vi "Auto Play Path.vi"(8 "Operation":T1, 9 "Auto Data":T13, 10 "Motors":T2 {"Radii (ft)"."Right Back Position" format="%.2f"; "Radii (ft)"."Right Front Position" format="%.2f"; "Radii (ft)"."Left Back Position" format="%.2f"; "Radii (ft)"."Left Front Position" format="%.2f"; "Pigeon2"."Type" items=["CAN"=352321536, "TalonSRX"=33554432]}) -> (0 "Auto Done?":bool)   [LabVIEW 2023]
uses:
  swerve-template/Type Definitions/Data/Robot Velocities.ctl
  swerve-template/Type Definitions/Hardware/Swerve Drives/(NEO-NEO-ThroughBore-Pigeon2) Swerve.ctl
  swerve-template/Type Definitions/Hardware/4 Motor Sets/(NEO & NEO 550) 4 Motor Set.ctl
  <vilib>/Rock Robotics/WPI/MotorControl/WPI_MotorControlDeviceRef.ctl
  <vilib>/Rock Robotics/WPI/MotorControl/WPI_MotorControlType.ctl
  <vilib>/Rock Robotics/SystemInterfaces/DIO/FPGA_DIOPWMChannel.ctl
  <vilib>/Rock Robotics/WPI/PWM/WPI_PWMDeadband.ctl
  <vilib>/Rock Robotics/SystemInterfaces/DIO/FPGA_DIOChannel.ctl
  <vilib>/Rock Robotics/WPI/ThirdParty/Phoenix-LabVIEW/Pigeon IMU/CTRE_PigeonIMU_DeviceRef.ctl
  <vilib>/Rock Robotics/WPI/ThirdParty/Phoenix-LabVIEW/Pigeon IMU/CTRE_PigeonIMU_ConnectionType.ctl
  swerve-template/Type Definitions/Data/Pod Positions.ctl
  Implementation/Drive Operations.ctl
  <vilib>/Platform/TimedLoop/XDataNode/timing_clust.ctl
  <vilib>/Platform/TimedLoop/XDataNode/nitl_modes.ctl
  <vilib>/Platform/TimedLoop/XDataNode/wakeup.ctl
  <vilib>/Rock Robotics/WPI/ThirdParty/REV Robotics/REVLib/Typedef/Spark MAX Control Type.ctl
  <vilib>/Rock Robotics/WPI/DriverStation/WPI_DriverStationRobotMode2.ctl
  <vilib>/Rock Robotics/Network Tables/NT Read Boolean.vi
  Framework/Robot Global Data.vi
  <vilib>/Platform/TimedLoop/XDataNode/XDataNode.xnode
  <vilib>/Platform/TimedLoop/XDataNode/XDNodeRunTimeDep.lvlib
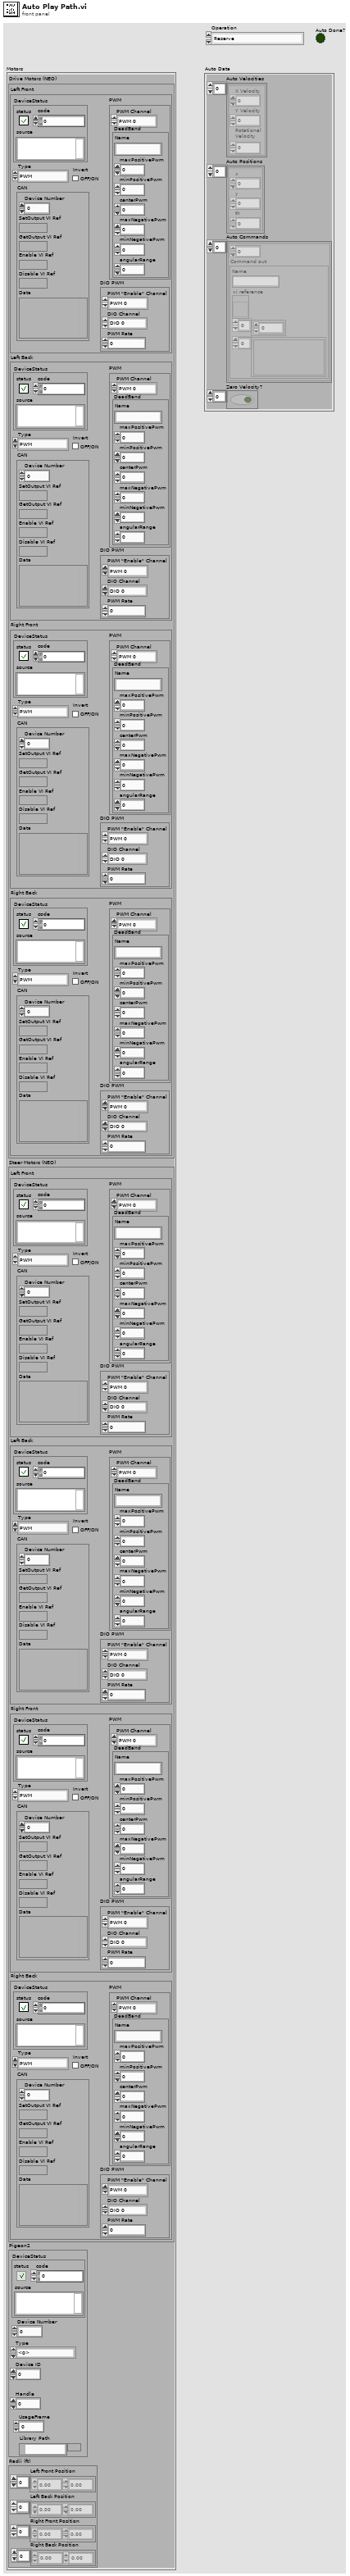
[diagram p1: front panel]
types:
  T1 = typedef "Drive Operations.ctl" = enum16{"Reserve", "Read Current", "Immediate", "Calibrate", "Auto"}
  T2 = typedef "(NEO-NEO-ThroughBore-Pigeon2) Swerve.ctl" = cluster{"Drive Motors (NEO)":T3, "Steer Motors (NEO)":T3, "Pigeon2":T9, "Radii (ft)":T11}
  T3 = typedef "(NEO & NEO 550) 4 Motor Set.ctl" = cluster{"Left Front":T4, "Left Back":T4, "Right Front":T4, "Right Back":T4}
  T4 = typedef "WPI_MotorControlDeviceRef.ctl" = cluster{"DeviceStatus":errorcluster, "Type":T5, "PWM":cluster{"PWM Channel":T6, "DeadBand":T7}, "CAN":cluster{"Device Number":u8, "SetOutput VI Ref":variant, "GetOutput VI Ref":variant, "Enable VI Ref":variant, "Disable VI Ref":variant, "Data":variant}, "Invert":bool, "DIO PWM":cluster{"PWM \"Enable\" Channel":T6, "DIOChannel":T8, "PWM Rate":dbl}}
  T5 = typedef "WPI_MotorControlType.ctl" = enum16{"PWM", "CAN", "DIO PWM"}
  T6 = typedef "FPGA_DIOPWMChannel.ctl" = enum8{"PWM 0", "PWM 1", "PWM 2", "PWM 3", "PWM 4", "PWM 5", "PWM 6", "PWM 7", "PWM 8", "PWM 9", "PWM MXP 0", "PWM MXP 1", "PWM MXP 2", "PWM MXP 3", "PWM MXP 4", "PWM MXP 5", "PWM MXP 6", "PWM MXP 7", "PWM MXP 8", "PWM MXP 9", "Invalid"}
  T7 = typedef "WPI_PWMDeadband.ctl" = cluster{"Name":string, "maxPositivePwm":i32, "minPositivePwm":i32, "centerPwm":i32, "maxNegativePwm":i32, "minNegativePwm":i32, "angularRange":u16}
  T8 = typedef "FPGA_DIOChannel.ctl" = enum8{"DIO 0", "DIO 1", "DIO 2", "DIO 3", "DIO 4", "DIO 5", "DIO 6", "DIO 7", "DIO 8", "DIO 9", "DIO MXP 0", "DIO MXP 1", "DIO MXP 2", "DIO MXP 3", "DIO MXP 4", "DIO MXP 5", "DIO MXP 6", "DIO MXP 7", "DIO MXP 8", "DIO MXP 9", "DIO MXP 10", "DIO MXP 11", "DIO MXP 12", "DIO MXP 13", "DIO MXP 14", "DIO MXP 15", "SPI Port CS1", "SPI Port CS2", "SPI Port CS3", "SPI Port MISO", "SPI Port MOSI", "Invalid"}
  T9 = typedef "CTRE_PigeonIMU_DeviceRef.ctl" = cluster{"DeviceStatus":errorcluster, "Device Number":u8, "Type":T10, "Device ID":u32, "Handle":u64, "UsageFrame":u32, "Library Path":path}
  T10 = typedef "CTRE_PigeonIMU_ConnectionType.ctl" = u32
  T11 = typedef "Pod Positions.ctl" = cluster{"Left Front Position":dbl[], "Left Back Position":dbl[], "Right Front Position":dbl[], "Right Back Position":dbl[]}
  T12 = typedef "Robot Velocities.ctl" = cluster{"X Velocity":dbl, "Y Velocity":dbl, "Rotational \nVelocity":dbl}
  T13 = cluster{"Auto Velocities":T12[], "Auto Positions":cluster{"x":dbl, "y":dbl, "th":dbl}[], "Auto Commands":cluster{dbl, "Command out":cluster{"Name":string, "vi reference":refnum<vi>, i32[], variant[]}}[], "Zero Velocity?":bool[]}
  T14 = cluster{"Time (s)":dbl, "Command out":cluster{"Name":string, "vi reference":refnum<vi>, i32[], variant[]}}
  T15 = typedef "Spark MAX Control Type.ctl" = enum16{"Percent VBus", "Voltage", "Velocity", "Position", "Smart Motion", "Current", "Smart Velocity", "MAXMotion Position", "MAXMotion Velocity"}
  T16 = cluster{"Left Front":dbl, "Left Back":dbl, "Right Front":dbl, "Right Back":dbl}
  T17 = typedef "XDNodeRunTimeDep.lvlib/timing_clust.ctl" = cluster{"Expected End [f-1]":u64, "Actual End [f-1]":u64, "Finished Late? [f-1]":bool, "Expected End [i-1]":u64, "Actual End [i-1]":u64, "Finished Late? [i-1]":bool, "Expected Start [i]":u64, "Actual Start [i]":u64, "Expected Start [f]":u64, "Actual Start [f]":u64, "Source Name":string, "Structure Name":string, "Period":i64, "Deadline":i64, "Offset":i64, "Start":i64, "Priority":i32, "Timeout":i32, "Mode":T18, "Wakeup Reason":T19, "Error":errorcluster, "Source Type":string, "Secondary Source Type":string, "Global End Time":u64, "Global Start Time":u64, "Frame Duration":u64, "Iteration Duration":u64, "Assigned CPU":i32, "I/O Scan Engine Mode":u32}
  T18 = typedef "XDNodeRunTimeDep.lvlib/nitl_modes.ctl" = enum32{"No Change", "Process missed periods, maintain original phase", "Discard missed periods, maintain original phase", "Process missed periods, ignore original phase", "Discard missed periods, ignore original phase"}
  T19 = typedef "XDNodeRunTimeDep.lvlib/wakeup.ctl" = enum32{"Normal", "Aborted", "Asynchronous wakeup", "Timing source error", "Timed loop error", "Timeout"}
  T20 = cluster{dbl, "Command out":cluster{"Name":string, "vi reference":refnum<vi>, i32[], variant[]}}[]
  T21 = typedef "WPI_DriverStationRobotMode2.ctl" = enum16{"Autonomous Disabled", "Autonomous Enabled", "Teleop Disabled", "Teleop Enabled", "Disconnected", "Finish", "Test Disabled", "Test Enabled", "Emergency Stopped"}
  T22 = cluster{dbl, "Y Velocity":dbl, "Rotational \nVelocity":dbl}
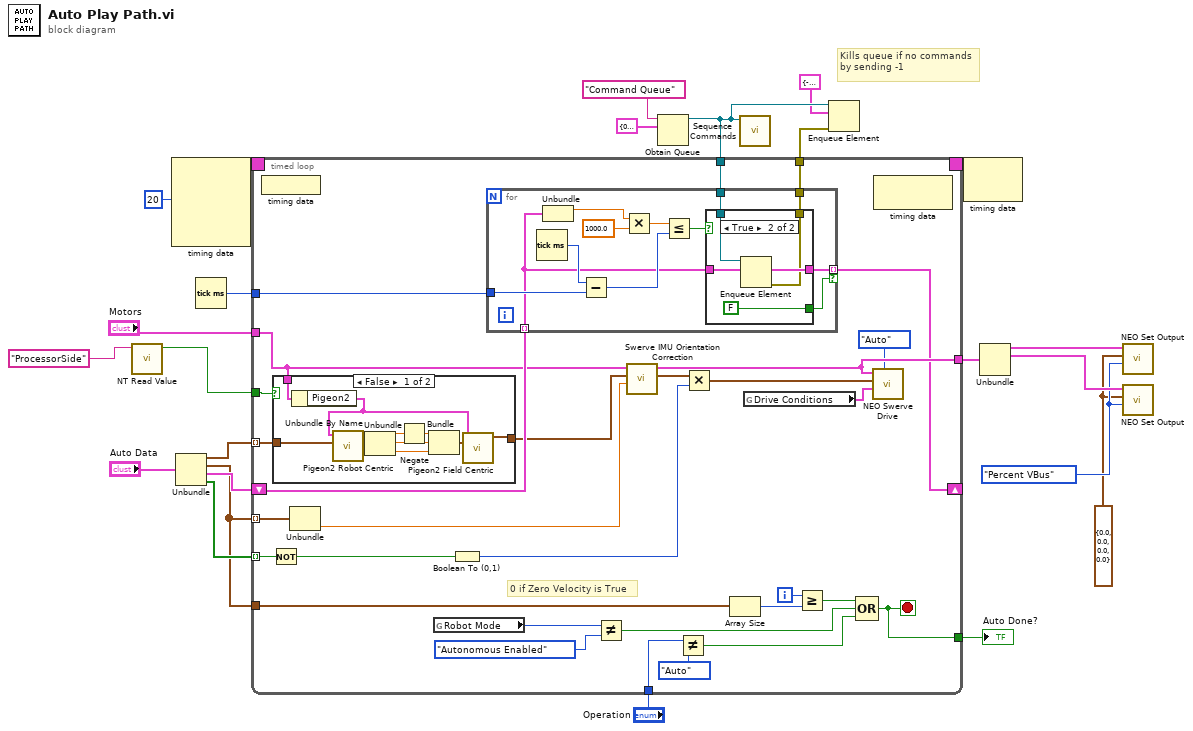
[diagram p0: block diagram]
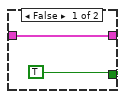
[diagram p3: hidden frame]
diagram:
  w9 = Spark_MAX_Control_Type."Percent VBus" ("Control Mode")
  w8 = T16 {"Left Front"=0.0, "Left Back"=0.0, "Right Front"=0.0, "Right Back"=0.0} ("Setpoints")
  # "Kills queue if no commands by sending -1"
  n1 = call-poly <vilib>:"NT Read Value.vi"("name"="ProcessorSide") -> ("value"=w2:bool)  [unwired: 8 in, 2 out]
  n2 = node-c288(i64 20 ("Period")) -> (w24:T17)  [unwired: 3 in]
  n3 = Unbundle("Auto Data") -> ("Auto Velocities"=w17:T12[], "Auto Positions"=w18:cluster{"x":dbl, "y":dbl, "th":dbl}[], "Auto Commands"=w20:T20, "Zero Velocity?"=w21:bool[])
  n4 = Tick Count (ms)() -> (millisecond timer value=w19:u32)
  n5 = Obtain Queue(name (unnamed)="Command Queue", element data type=T14 {"Time (s)"=0.0, "Command out"={"Name"="", "vi reference"=refnum, [], []}} ("element")) -> (queue out=w5:refnum<queue>)  [unwired: 3 in, 2 out]
  n6 = timed-loop {
    timing: w24 -> [_]
    timing-out: [_] -> w23
    tunnel: "Motors" -> [w25]
    tunnel: [w52] -> w7
    tunnel: w17 -> [w28] mode=indexing
    tunnel: w18 -> [w51] mode=indexing
    tunnel: w18 -> [w50]
    tunnel: w19 -> [w49]
    tunnel: w5 -> [w47]
    shift-right: [w45] -> _
    shift-left: w20 -> [w44]
    tunnel: w21 -> [w34] mode=indexing
    tunnel: [w37] -> w22
    tunnel: "Operation" -> [w33]
    tunnel: [w32] -> w4
    tunnel: w2 -> [w26]
    i -> [w53]
    stop <- w37 stop-if-true
    # "0 if Zero Velocity is True"
    n7 = node-c288() -> ()  [unwired: 1 in]
    n8 = Not(x=w34) -> (.not. x?=w41:bool)
    n9 = case shown="False" w26 {
      tunnel: w28 -> [w64 w65]
      tunnel: [w63 w65] -> w27
      tunnel: w25 -> [w56 _]
      frame False {
        n10 = Unbundle By Name(w56) -> ("Pigeon2"=w55:T9)
        n11 = call "Pigeon2 Robot Centric.vi"("Robot Centric Velocities"=w64, "PigeonIMUDevRef"=w55) -> ("Field Centric Velocities"=w62:T12)  [unwired: 9 in]
        n12 = Unbundle(w62) -> ("X Velocity"=w61:dbl, "Y Velocity"=w59:dbl, "Rotational \nVelocity"=w58:dbl)
        n13 = Negate(x=w61) -> (-x=w60:dbl)
        n14 = Bundle(w60, "Y Velocity"=w59, "Rotational \nVelocity"=w58) -> (w57:T22)  [unwired: 1 in]
        n15 = call "Pigeon2 Field Centric.vi"("Field Centric Velocities"=w57, "PigeonIMUDevRef"=w55) -> ("Robot Centric Velocities"=w63:T12)  [unwired: 9 in]
      }
      frame True {
      }
    }
    n16 = Unbundle(w51) -> ("th"=w29:dbl)  [unwired: 2 out]
    n17 = global read "Robot Global Data.vi" "Robot Mode"() -> (w43:T21)
    n18 = Boolean To (0,1)(Boolean=w41) -> (0, 1=w40:i16)
    n19 = for {
      tunnel: w49 -> [w76]
      tunnel: w47 -> [w70]
      tunnel: w44 -> [w67] mode=indexing
      tunnel: [w69] -> w45 mode=indexing if=w68
      tunnel: [w66] -> w32
      n20 = Tick Count (ms)() -> (millisecond timer value=w77:u32)
      n21 = Unbundle(w67) -> (w75:dbl)  [unwired: 1 out]
      n22 = Subtract(x=w77, y=w76) -> (x-y=w72:u32)
      n23 = Multiply(x=w75, y=1000.0) -> (x*y=w73:dbl)
      n24 = Less Or Equal?(x=w73, y=w72) -> (x <= y?=w71:bool)
      n25 = case shown="True" w71 {
        tunnel: w70 -> [_ w83]
        tunnel: w67 -> [w78 w82]
        tunnel: [w78 w82] -> w69
        tunnel: [TRUE FALSE] -> w68
        tunnel: [_ w80] -> w66
        frame False {
        }
        frame True {
          n26 = Enqueue Element(queue=w83, element=w82) -> (error out=w80:errorcluster)  [unwired: 2 in, 2 out]
        }
      }
    }
    n27 = Not Equal?(x=w43, y=WPI_DriverStationRobotMode2."Autonomous Enabled") -> (x != y?=w38:bool)
    n28 = call "Swerve IMU Orientation Correction.vi"("Setpoint"=w29, "Robot Velocities In"=w27, "Motors In"=w25) -> ("Robot Velocities Out"=w31:T12, "Motors Out"=w52:T2)  [unwired: 7 in]
    n29 = Not Equal?(x=w33, y=Drive_Operations."Auto") -> (x != y?=w36:bool)
    n30 = Multiply(x=w31, y=w40) -> (x*y=w39:T12)
    n31 = Array Size(array=w50) -> (size(s)=w54:i32)
    n32 = global read "Robot Global Data.vi" "Drive Conditions"() -> (w30:cluster{"Field Centric":bool})
    n33 = Greater Or Equal?(x=w53, y=w54) -> (x >= y?=w48:bool)
    n34 = Compound Arithmetic op=OR(w48, w38, w36) -> (w37:bool)
    n35 = call "NEO Swerve Drive.vi"("Operation"=Drive_Operations."Auto", "Drive Conditions"=w30, "Robot Velocities"=w39, "Swerve Drive"=w52) -> ()  [unwired: 7 in, 1 out]
    n36 = node-c288() -> ()  [unwired: 1 in, 1 out]
  }
  "Auto Done?" <- w22
  n37 = call "Sequence Commands.vi"("queue in"=w5) -> ()  [unwired: 11 in]
  n38 = Enqueue Element(queue=w5, element=T14 {"Time (s)"=-1.0, "Command out"={"Name"="", "vi reference"=refnum, [], []}}, error in (no error)=w4) -> ()  [unwired: 1 in, 3 out]
  n39 = node-c288(w23) -> ()  [unwired: 1 out]
  n40 = Unbundle(w7) -> ("Drive Motors (NEO)"=w11:T3, "Steer Motors (NEO)"=w10:T3)  [unwired: 2 out]
  n41 = call "NEO Set Output.vi"("Control Mode"=w9, "Setpoints"=w8, "Motors"=w11) -> ()  [unwired: 9 in]
  n42 = call "NEO Set Output.vi"("Control Mode"=w9, "Setpoints"=w8, "Motors"=w10) -> ()  [unwired: 9 in]
